vi "DOCK_PRINTER_read_template.vi"(7 "error_in":errorcluster) -> (0 "error_out":errorcluster, 3 "label":string)   [LabVIEW 2019]
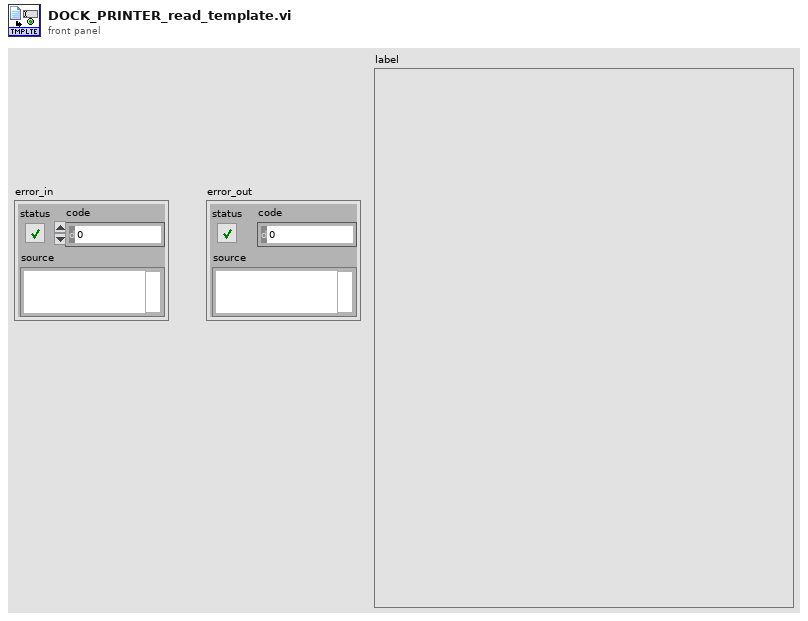
[diagram p1: front panel]
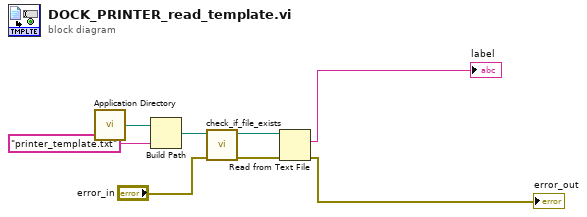
[diagram p0: block diagram]
diagram:
  n1 = call <vilib>:"Application Directory.vi"() -> ("Application Directory"=w8:path)
  n2 = Build Path(base path=w8, name or relative path="printer_template.txt") -> (appended path=w6:path)
  n3 = call "check_if_file_exists.vi"("error_in"="error_in", "file_path_in"=w6) -> ("error_out"=w5:errorcluster, "file_path_out"=w4:path)  [unwired: 8 in]
  n4 = Read from Text File(file (use dialog)=w4, error in=w5) -> (text=→"label":string, error out=→"error_out":errorcluster)  [unwired: 2 in, 2 out]
